vi "站点信息设置.vi"() -> ()   [LabVIEW 2016]
uses:
  <vilib>/Utility/miscctls.llb/LVPointTypeDef.ctl
  <vilib>/Utility/config.llb/NI_LVConfig.lvlib
panel:
  in  "站点系列号":string
  in  "站点名称":string
  in  "布尔":bool
  in  "取消":bool
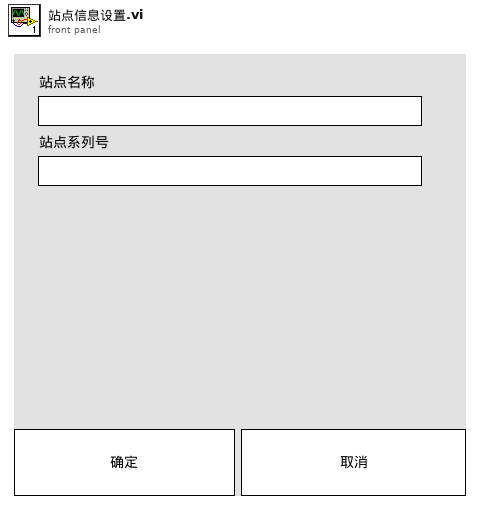
[diagram p1: front panel]
types:
  T1 = typedef "LVPointTypeDef.ctl" = cluster{"Horizontal":i16, "Vertical":i16}
  T2 = typedef "NI_LVConfig.lvlib/Config Data RefNum.ctl" = refnum<k1>
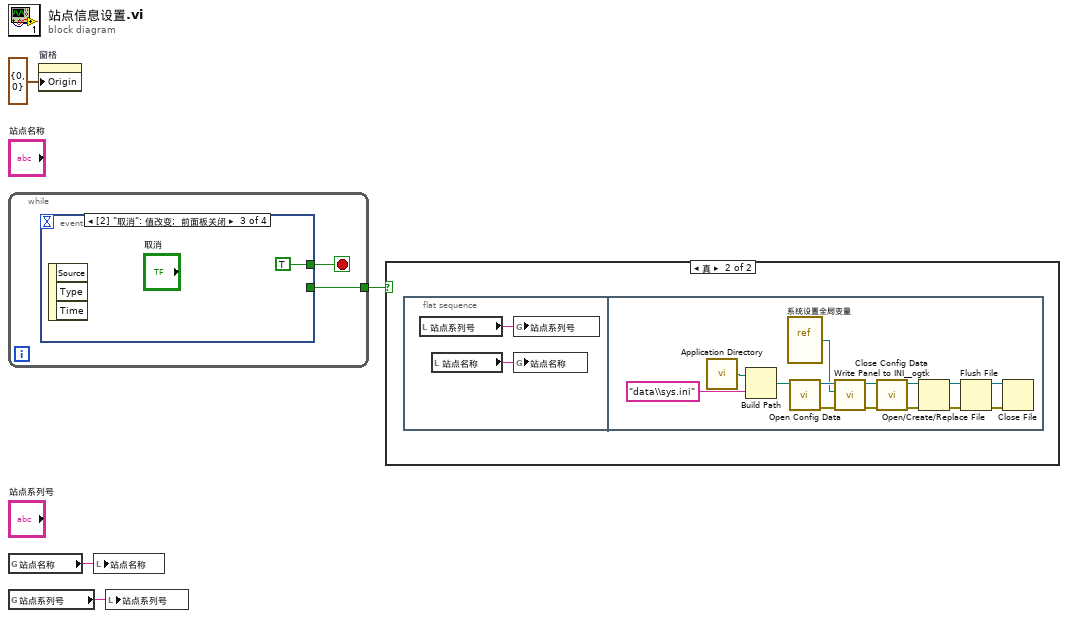
[diagram p0: block diagram]
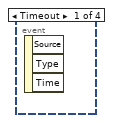
[diagram p3: hidden frame]
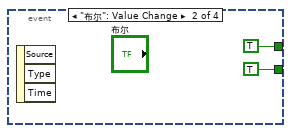
[diagram p4: hidden frame]
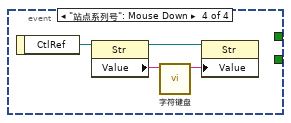
[diagram p5: hidden frame]
diagram:
  n1 = while {
    tunnel: [w5] -> w1
    stop <- w6 stop-if-true
    n2 = event shown="[2] \"取消\": 值改变;  前面板关闭" {
      selector: _ -> [_ _ _ _]
      dyn-events: _ -> [_ _ _ _]
      timeout: _ -> [_ _ _ _]
      tunnel: [_ TRUE TRUE _] -> w6
      tunnel: [_ TRUE _ _] -> w5
      event Timeout {
        n3 = event-data() -> ()  [unwired: 1 in, 3 out]
      }
      event "布尔": Value Change {
        n4 = event-data() -> ()  [unwired: 1 in, 3 out]
      }
      event "取消": Value Change; Panel Close {
        n5 = event-data() -> ()  [unwired: 1 in, 3 out]
      }
      event "站点系列号": Mouse Down {
        n6 = event-data() -> ("CtlRef"=w13:refnum<vi>)  [unwired: 1 in]
        n7 = property class="Str"(reference=w13) -> (reference out=w10:refnum<vi>, "Value"=w12:string)  [unwired: 1 in, 1 out]
        n8 = call "字符键盘.vi"("Old String"=w12) -> ("String"=w11:string)  [unwired: 10 in]
        n9 = property class="Str"(reference=w10, "Value"=w11) -> ()  [unwired: 1 in, 2 out]
      }
    }
  }
  n10 = global read "系统设置全局变量.vi" "站点名称"() -> (w3:string)
  n11 = global read "系统设置全局变量.vi" "站点系列号"() -> (w2:string)
  n12 = property on="窗格" class="Pane"("Origin"=T1 {"Horizontal"=0, "Vertical"=0} ("原点")) -> ()  [unwired: 2 in, 2 out]
  n13 = local write "站点名称"(w3) -> ()
  n14 = local write "站点系列号"(w2) -> ()
  n15 = case shown="真" w1 {
    frame False {
    }
    frame True {
      n16 = flat-sequence {
        frame #0 {
          n17 = local read "站点系列号"() -> (w15:string)
          n18 = local read "站点名称"() -> (w14:string)
          n19 = global write "系统设置全局变量.vi" "站点系列号"(w15) -> ()
          n20 = global write "系统设置全局变量.vi" "站点名称"(w14) -> ()
        }
        frame #1 {
          n21 = call <vilib>:"Application Directory.vi"() -> ("Application Directory"=w29:path)
          n22 = Build Path(base path=w29, name or relative path="data\\sys.ini" ("名称或相对路径")) -> (appended path=w27:path)
          n23 = vi-ref "系统设置全局变量.vi"() -> (w25:refnum<vi>)
          n24 = call <vilib>:"Open Config Data.vi"("configuration file path"=w27) -> ("error out"=w23:errorcluster, "refnum"=w26:T2)  [unwired: 8 in, 1 out]
          n25 = call <userlib>:"Write Panel to INI__ogtk.vi"("error in (no error)"=w23, "VI ref"=w25, "refnum"=w26) -> ("error out"=w22:errorcluster, "refnum out"=w24:T2)  [unwired: 7 in]
          n26 = call <vilib>:"Close Config Data.vi"("error in (no error)"=w22, "refnum"=w24) -> ("error out"=w17:errorcluster, "file path"=w16:path)  [unwired: 8 in]
          n27 = Open/Create/Replace File(file path (use dialog)=w16, error in=w17) -> (refnum out=w20:refnum<file>, error out=w21:errorcluster)  [unwired: 4 in, 1 out]
          n28 = Flush File(refnum=w20, error in=w21) -> (refnum out=w19:refnum<file>, error out=w18:errorcluster)
          n29 = Close File(refnum=w19, error in=w18) -> ()  [unwired: 2 out]
        }
      }
    }
  }
